vi "UpdateModeID.vi"(10 "Mode IDs":string[](array[string]), 11 "Array in":T1[](array[typedef]) {"Modes"."Amplititute" step=0.05}) -> (3 "Array out":T1[](array[typedef]) {"Modes"."Amplititute" step=0.05})   [LabVIEW 2014]
uses:
  Controls/Holo Settings.ctl
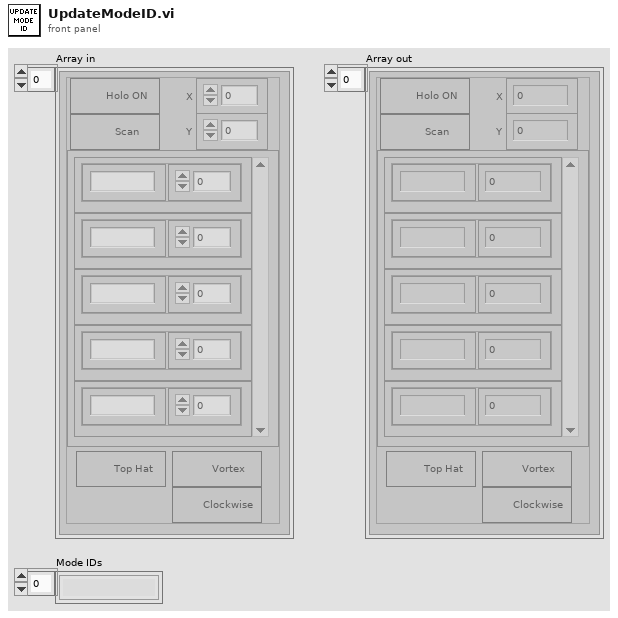
[diagram p1: front panel]
types:
  T1 = typedef "Holo Settings.ctl" = cluster{"Top Hat":bool, "Modes":cluster{"Mode ID":string, "Amplititute":dbl}[], "Vortex":bool, "Clockwise":bool, "X":dbl, "Y":dbl, "Holo ON":bool, "Scan":bool}
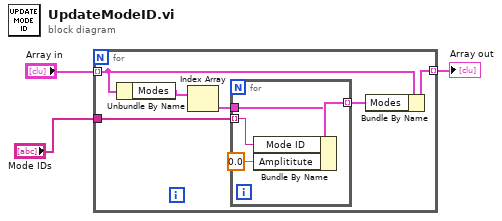
[diagram p0: block diagram]
diagram:
  n1 = for {
    tunnel: "Array in" -> [w8] mode=indexing
    tunnel: "Mode IDs" -> [w9]
    tunnel: [w6] -> w2 mode=indexing
    n2 = Unbundle By Name(w8) -> ("Modes"=w5:cluster{"Mode ID":string, "Amplititute":dbl}[])
    n3 = Index Array(array=w5) -> (element=w4:cluster{"Mode ID":string, "Amplititute":dbl})  [unwired: 1 in]
    n4 = for {
      tunnel: w9 -> [w13] mode=indexing
      tunnel: [w12] -> w7 mode=indexing
      tunnel: w4 -> [w11]
      n5 = Bundle By Name(cluster=w11, "Mode ID"=w13, "Amplititute"=0.0) -> (w12:cluster{"Mode ID":string, "Amplititute":dbl})
    }
    n6 = Bundle By Name(cluster=w8, "Modes"=w7) -> (w6:T1)
  }
  "Array out" <- w2
